vi "Initialize_Power_Supplies.vi"() -> (0 "error out":errorcluster, 1 "Available Power Supplies":T1)   [LabVIEW 2020]
uses:
  <vilib>/Instr/_visa.llb/VISA Open Access Mode.ctl
  <vilib>/Utility/file.llb/Read Delimited Spreadsheet (string).vi
panel:
  out "Power Supplies from file":T2
  out "List of Found Power Supply Addresses":string[](array[string])
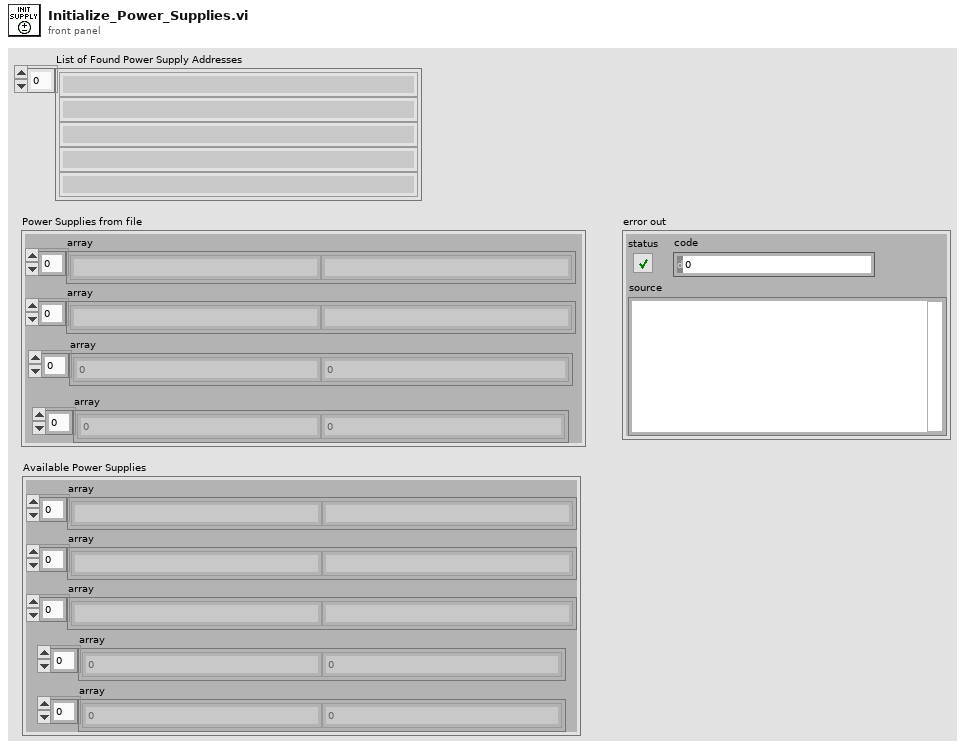
[diagram p1: front panel]
types:
  T1 = cluster{"array":string[], "array":string[], "array":string[], "array":dbl[], "array":dbl[]}
  T2 = cluster{"array":string[], "array":string[], "array":dbl[], "array":dbl[]}
  T3 = typedef "VISA Open Access Mode.ctl" = u32
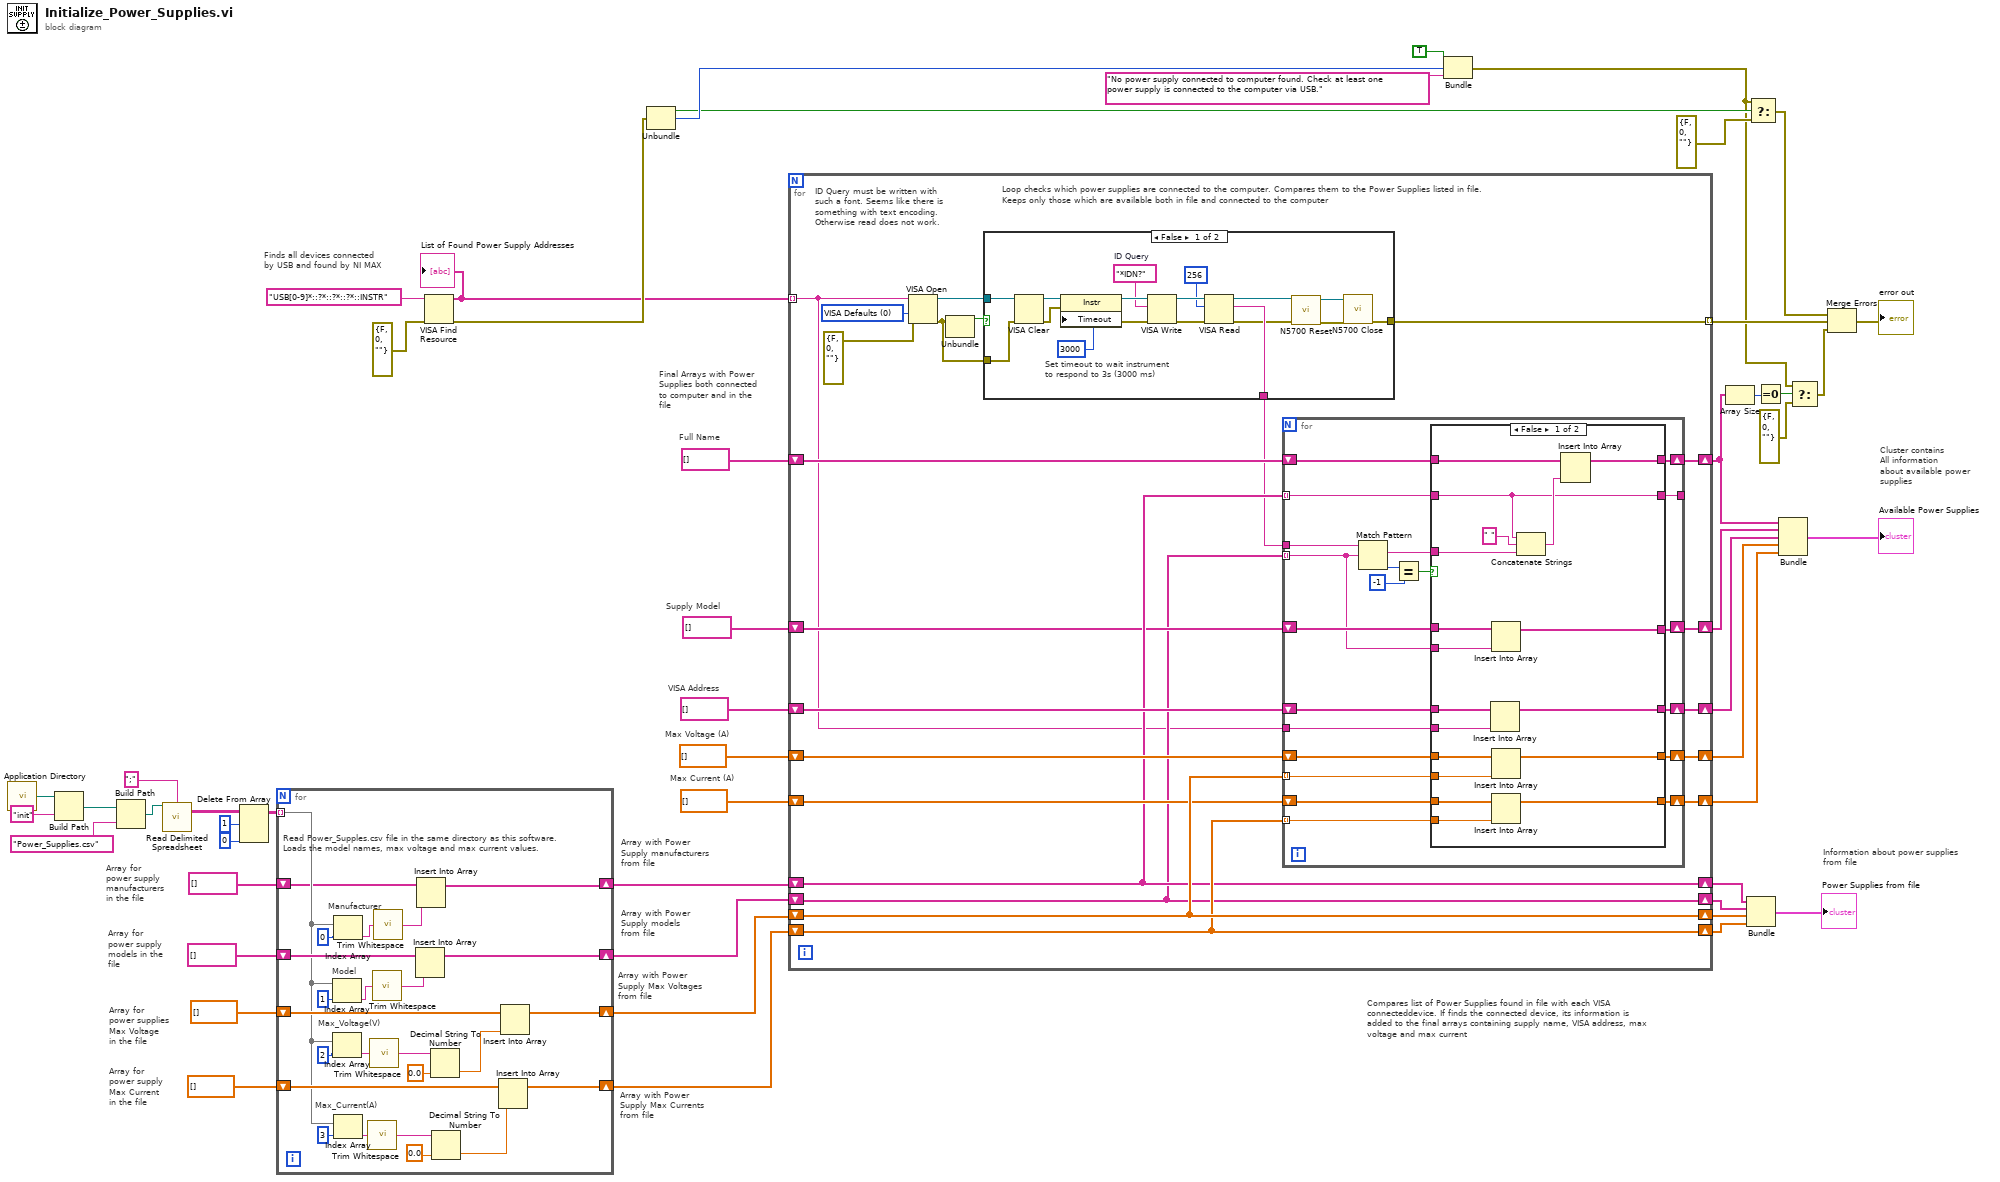
[diagram p0: block diagram]
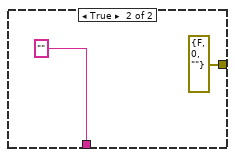
[diagram p2: hidden frame]
diagram:
  # "Compares list of Power Supplies found in file with each VISA connecteddevice. If finds the connected device, its information is added to the final arrays containing supply name, VISA address, max voltage and max current"
  # "Supply Model"
  # "Array with Power\nSupply manufacturers\nfrom file"
  # "Array for \npower supply\nmanufacturers\nin the file"
  # "Information about power supplies\nfrom file"
  # "Full Name"
  # "VISA Address"
  # "Max Voltage (A)"
  # "Max Current (A)"
  # "Array with Power\nSupply Max Currents \nfrom file"
  # "Array with Power\nSupply Max Voltages \nfrom file"
  # "Array with Power\nSupply models\nfrom file"
  # "Final Arrays with Power\nSupplies both connected\nto computer and in the \nfile"
  # "Cluster contains\nAll information \nabout available power \nsupplies"
  # "Array for \npower supply\nMax Current\nin the file"
  # "Array for \npower supplies\nMax Voltage\nin the file"
  # "Array for \npower supply\nmodels in the \nfile"
  # "Finds all devices connected \nby USB and found by NI MAX"
  n1 = call <vilib>:"Application Directory.vi"() -> ("Application Directory"=w25:path)
  n2 = Build Path(base path=w25, name or relative path="init") -> (appended path=w24:path)
  n3 = Build Path(base path=w24, name or relative path="Power_Supplies.csv") -> (appended path=w50:path)
  n4 = call-poly <vilib>:"Read Delimited Spreadsheet.vi"("file path (dialog if empty)"=w50, "delimiter (\\t)"=";" ("delimiter (\\t)")) -> ("all rows"=w49:string[][])  [unwired: 8 in, 5 out]
  n5 = Delete From Array(array=w49, length=1, index (row)=0) -> (array with subset deleted=w46:string[][])  [unwired: 1 in, 1 out]
  n6 = for {
    tunnel: w46 -> [w57] mode=indexing
    shift-right: [w64] -> w42
    shift-left: string[] [] ("array") -> [w65]
    shift-right: [w59] -> w36
    shift-left: dbl[] [] ("array") -> [w60]
    shift-right: [w58] -> w41
    shift-left: dbl[] [] ("array") -> [w61]
    shift-right: [w52] -> w29
    shift-left: string[] [] ("array") -> [w53]
    # "Read Power_Supples.csv file in the same directory as this software.\nLoads the model names, max voltage and max current values."
    # "Manufacturer"
    # "Max_Current(A)"
    # "Max_Voltage(V)"
    # "Model"
    n7 = Index Array(array=w57, index=1) -> (element=w72:string)
    n8 = Index Array(array=w57, index=2) -> (element=w73:string)
    n9 = Index Array(array=w57, index=0) -> (element=w55:string)
    n10 = Index Array(array=w57, index=3) -> (element=w70:string)
    n11 = call <vilib>:"Trim Whitespace.vi"("string"=w70) -> ("trimmed string"=w69:string)  [unwired: 1 in]
    n12 = call <vilib>:"Trim Whitespace.vi"("string"=w73) -> ("trimmed string"=w71:string)  [unwired: 1 in]
    n13 = call <vilib>:"Trim Whitespace.vi"("string"=w72) -> ("trimmed string"=w66:string)  [unwired: 1 in]
    n14 = call <vilib>:"Trim Whitespace.vi"("string"=w55) -> ("trimmed string"=w54:string)  [unwired: 1 in]
    n15 = Insert Into Array(array=w65, new element=w66) -> (w64:string[])  [unwired: 1 in]
    n16 = Insert Into Array(array=w53, new element=w54) -> (w52:string[])  [unwired: 1 in]
    n17 = Decimal String To Number(string=w71, default (0L)=0.0) -> (number=w63:dbl)  [unwired: 1 in, 1 out]
    n18 = Decimal String To Number(string=w69, default (0L)=0.0) -> (number=w62:dbl)  [unwired: 1 in, 1 out]
    n19 = Insert Into Array(array=w60, new element=w62) -> (w59:dbl[])  [unwired: 1 in]
    n20 = Insert Into Array(array=w61, new element=w63) -> (w58:dbl[])  [unwired: 1 in]
  }
  n21 = VISA Find Resource(8:errorcluster {"status"=FALSE, "code"=0, "source"=""} ("error in (no error)"), 11:"USB[0-9]*::?*::?*::?*::INSTR" ("expression (\"?*\")")) -> (0:w31:errorcluster, 3:w15:string[])  [unwired: 1 in, 1 out]
  "List of Found Power Supply Addresses" <- w15
  n22 = Unbundle(w31) -> ("status"=w4:bool, "code"=w5:i32)  [unwired: 1 out]
  n23 = for {
    shift-right: [w84] -> w35
    shift-left: w42 -> [w84]
    shift-right: [w97] -> w34
    shift-left: w41 -> [w97]
    shift-right: [w96] -> w33
    shift-left: w36 -> [w96]
    shift-right: [w88] -> w18
    shift-left: dbl[] [] ("array") -> [w95]
    shift-right: [w89] -> w19
    shift-left: dbl[] [] ("array") -> [w94]
    shift-right: [w90] -> w20
    shift-left: string[] [] ("array") -> [w93]
    shift-right: [w91] -> w12
    shift-left: string[] [] ("array") -> [w92]
    shift-right: [w87] -> w28
    shift-left: w29 -> [w87]
    shift-right: [w85] -> w21
    shift-left: string[] [] ("array") -> [w86]
    tunnel: w15 -> [w82] mode=indexing
    tunnel: [w77] -> w13 mode=indexing
    w98 = T3 0 items=["VISA Defaults"=0, "Exclusive Lock"=1, "Load Configured Settings"=4] ("Access Mode")
    # "Loop checks which power supplies are connected to the computer. Compares them to the Power Supplies listed in file. \nKeeps only those which are available both in file and connected to the computer"
    # "ID Query must be written with\nsuch a font. Seems like there is \nsomething with text encoding. \nOtherwise read does not work."
    n24 = VISA Open(access mode=w98, error in (no error)=errorcluster {"status"=FALSE, "code"=0, "source"=""}, VISA resource name=w82) -> (VISA resource name=w80:refnum<visa-resource-name>, error out=w79:errorcluster)  [unwired: 2 in]
    n25 = Unbundle(w79) -> ("status"=w81:bool)  [unwired: 2 out]
    n26 = case shown="False" w81 {
      tunnel: w80 -> [w107 _]
      tunnel: w79 -> [w106 _]
      tunnel: [w104 "" ("read buffer")] -> w78
      tunnel: [w99 errorcluster {"status"=FALSE, "code"=0, "source"=""} ("error out")] -> w77
      frame False {
        w110 = "*IDN?"  # ID Query
        # "Set timeout to wait instrument \nto respond to 3s (3000 ms)"
        n27 = VISA Clear(VISA resource name=w107, error in (no error)=w106) -> (VISA resource name out=w112:refnum<visa-resource-name>, error out=w113:errorcluster)
        n28 = property class="Instr"(reference=w112, error in=w113, "Timeout"=u32 3000 ("General Settings:Timeout Value")) -> (reference out=w114:refnum<visa-resource-name>, error out=w115:errorcluster)
        n29 = VISA Write(VISA resource name=w114, write buffer=w110, error in (no error)=w115) -> (VISA resource name out=w111:refnum<visa-resource-name>, error out=w105:errorcluster)  [unwired: 1 out]
        n30 = VISA Read(VISA resource name=w111, byte count=u32 256, error in (no error)=w105) -> (VISA resource name out=w101:refnum<visa-resource-name>, read buffer=w104:string, error out=w100:errorcluster)  [unwired: 1 out]
        n31 = call "N5700 Reset.vi"("error"=w100, "VISA"=w101) -> ("error out"=w103:errorcluster, "VISA out"=w102:refnum<visa-resource-name>)  [unwired: 5 in]
        n32 = call "N5700 Close.vi"("error"=w103, "VISA name"=w102) -> ("error out"=w99:errorcluster)  [unwired: 6 in]
      }
      frame True {
      }
    }
    n33 = for {
      tunnel: w84 -> [w118] mode=indexing
      tunnel: w78 -> [w133]
      tunnel: w97 -> [w135] mode=indexing
      tunnel: w96 -> [w134] mode=indexing
      shift-right: [w131] -> w88
      shift-left: w95 -> [w132]
      shift-right: [w129] -> w89
      shift-left: w94 -> [w130]
      shift-right: [w127] -> w90
      shift-left: w93 -> [w128]
      shift-right: [w125] -> w91
      shift-left: w92 -> [w126]
      tunnel: w82 -> [w123]
      tunnel: w87 -> [w122] mode=indexing
      tunnel: [w121] -> _
      shift-right: [w119] -> w85
      shift-left: w86 -> [w120]
      n34 = Match Pattern(string=w133, regular expression=w118) -> (match substring=w124:string, offset past match=w138:i32)  [unwired: 1 in, 2 out]
      n35 = Equal?(x=w138, y=-1) -> (x = y?=w136:bool)
      n36 = case shown="False" w136 {
        tunnel: w135 -> [w156 _]
        tunnel: w134 -> [w155 _]
        tunnel: w124 -> [w145 _]
        tunnel: w123 -> [w139 _]
        tunnel: w132 -> [w154 w159]
        tunnel: [w153 w159] -> w131
        tunnel: w130 -> [w152 w160]
        tunnel: [w151 w160] -> w129
        tunnel: w128 -> [w150 w162]
        tunnel: [w149 w162] -> w127
        tunnel: w126 -> [w148 w161]
        tunnel: [w147 w161] -> w125
        tunnel: w122 -> [w143 w158]
        tunnel: [w143 w158] -> w121
        tunnel: w120 -> [w142 w157]
        tunnel: [w141 w157] -> w119
        tunnel: w118 -> [w140 _]
        frame False {
          n37 = Insert Into Array(array=w150, new element=w139) -> (w149:string[])  [unwired: 1 in]
          n38 = Insert Into Array(array=w142, new element=w140) -> (w141:string[])  [unwired: 1 in]
          n39 = Insert Into Array(array=w152, new element=w156) -> (w151:dbl[])  [unwired: 1 in]
          n40 = Insert Into Array(array=w154, new element=w155) -> (w153:dbl[])  [unwired: 1 in]
          n41 = Concatenate Strings(w143, " " ("string"), w145) -> (w146:string)
          n42 = Insert Into Array(array=w148, new element=w146) -> (w147:string[])  [unwired: 1 in]
        }
        frame True {
        }
      }
    }
  }
  n43 = Bundle(TRUE, "code"=w5, "source"="No power supply connected to computer found. Check at least one power supply is connected to the computer via USB.") -> (w1:cluster{bool, "code":i32, "source":string})  [unwired: 1 in]
  n44 = Array Size(array=w12) -> (size(s)=w11:i32)
  n45 = Bundle("array"=w28, "array"=w35, "array"=w34, "array"=w33) -> (→"Power Supplies from file":T2)  [unwired: 1 in]
  n46 = Select(t=w1, s=w4, f=cluster{bool, "code":i32, "source":string} {FALSE, "code"=0, "source"=""}) -> (s? t:f=w2:cluster{bool, "code":i32, "source":string})
  n47 = Equal To 0?(x=w11) -> (x = 0?=w10:bool)
  n48 = Bundle("array"=w12, "array"=w21, "array"=w20, "array"=w19, "array"=w18) -> (→"Available Power Supplies":T1)  [unwired: 1 in]
  n49 = Select(t=w1, s=w10, f=errorcluster {"status"=FALSE, "code"=0, "source"=""}) -> (s? t:f=w8:errorcluster)
  n50 = Merge Errors(w2, w13, w8) -> (→"error out":errorcluster)
